vi "Define Parameter.vi"(8 "error in (no error)":errorcluster, 11 "Analyze q-Factor in":refnum<class "Analyze q-Factor.lvclass">) -> (0 "error out":errorcluster, 3 "Analyze q-Factor out":refnum<class "Analyze q-Factor.lvclass">)   [LabVIEW 2014, in "Analyze.lvlib" / "Analyze q-Factor.lvclass"]
uses:
  Analyze q-Factor.lvclass
  Analyze Parameter/Analyze Parameter Width Method/Width Method.lvclass
  Analyze Fluence/Analyze Fluence.lvclass
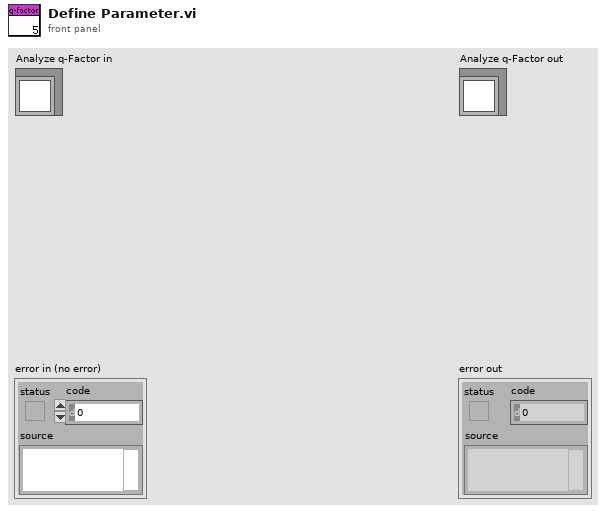
[diagram p1: front panel]
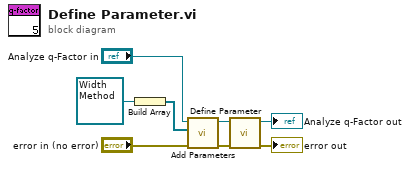
[diagram p0: block diagram]
diagram:
  n1 = Build Array(refnum<class "Width Method.lvclass"> refnum ("Width Method")) -> (w5:refnum<class "Width Method.lvclass">[])
  n2 = call-dynamic "Add Parameters.vi"("error in (no error)"="error in (no error)", "Parameters"=w5, "Analyze BaseClass in"="Analyze q-Factor in") -> ("error out"=w2:errorcluster, "Analyze BaseClass out"=w3:refnum<class "Analyze q-Factor.lvclass">)  [unwired: 7 in]
  n3 = call-parent "Define Parameter.vi"("error in (no error)"=w2, "Analyze Fluence in"=w3) -> ("error out"=→"error out":errorcluster, "Analyze Fluence out"=→"Analyze q-Factor out":refnum<class "Analyze q-Factor.lvclass">)  [unwired: 8 in]
